vi "Concat Strings Array.vi"(4 "Strings":refnum<class "Abs_Value.lvclass">[](array[class])) -> (1 "Result":refnum<class "Abs_String.lvclass">)   [LabVIEW 2021]
uses:
  Abs_Types/Value/Abs_Value.lvclass
  Abs_Types/String/Abs_String.lvclass
  Support/Concatenate/Concatenate_STR.lvclass
  C:/Program Files (x86)/National Instruments/LabVIEW 2021/vi.lib/TSA/Abstract Data Classes/Abs_Types/String/Abs_String.lvclass
  Support/Concatenate/Concatenate_STR.lvclass/Concatenate_STR.ctl
  Support/Concatenate/Properties/Write Strings.vi
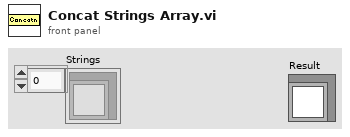
[diagram p1: front panel]
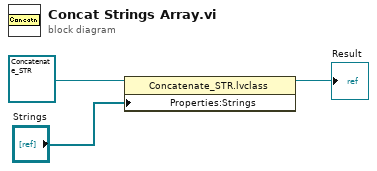
[diagram p0: block diagram]
diagram:
  n1 = property class="Concatenate_STR.lvclass"(reference=refnum<class "Concatenate_STR.lvclass"> refnum ("Concatenate_STR.lvclass"), "Properties:Strings"="Strings") -> (reference out=→"Result":refnum<class "Concatenate_STR.lvclass">)  [unwired: 1 in, 1 out]
